vi "Create_empty_waveform_file.vi"(11 "File#":u8) -> (0 "error out":errorcluster)   [LabVIEW 2017]
uses:
  <vilib>/Waveform/WDTFileIO.llb/ Write Waveform to File.vi
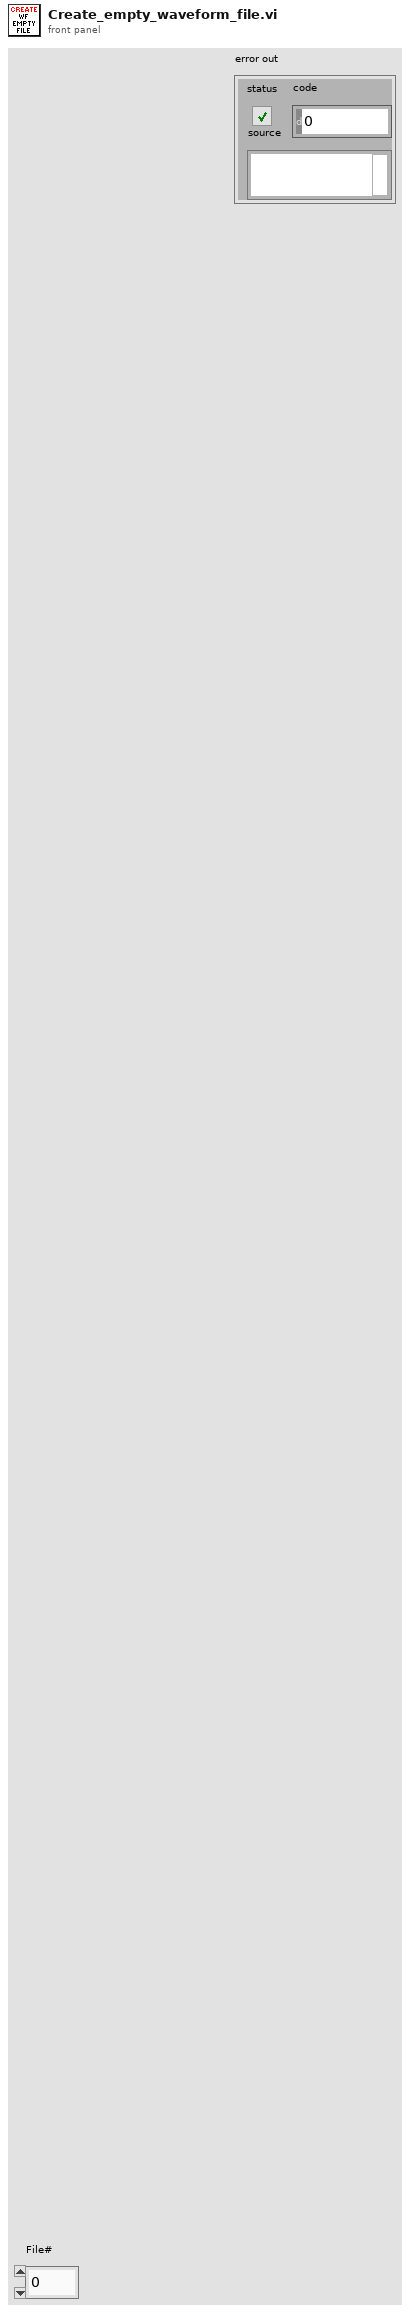
[diagram p1: front panel]
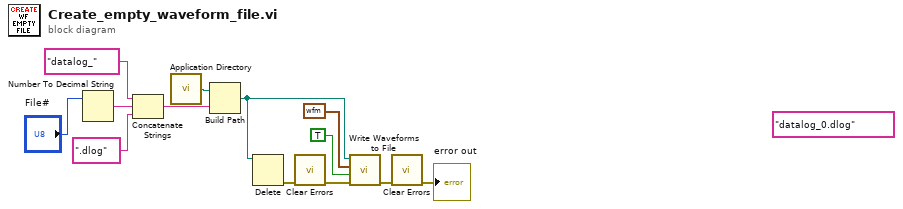
[diagram p0: block diagram]
diagram:
  (unwired) "datalog_0.dlog" ("pattern label")
  n1 = Number To Decimal String(number="File#") -> (decimal integer string=w4:string)  [unwired: 1 in]
  n2 = Concatenate Strings("datalog_" ("string"), w4, ".dlog" ("string")) -> (w3:string)
  n3 = call <vilib>:"Application Directory.vi"() -> ("Application Directory"=w6:path)
  n4 = Build Path(base path=w6, name or relative path=w3) -> (appended path=w11:path)
  n5 = Delete(path (use dialog)=w11) -> (error out=w9:errorcluster)  [unwired: 4 in, 2 out]
  n6 = call <vilib>:"Clear Errors.vi"("error in (no error)"=w9) -> ("error out"=w10:errorcluster)  [unwired: 5 in, 1 out]
  n7 = call-poly <vilib>:"Write Waveforms to File.vi"("error in (no error)"=w10, "append to file? (new file:F)"=TRUE, "waveform"=waveform(dbl) {"t0"=timestamp(0 s since 1904-01-01), "dt"=1.0, "Y"=[]}, "file path (dialog if empty)"=w11) -> ("error out"=w8:errorcluster)  [unwired: 6 in, 1 out]
  n8 = call <vilib>:"Clear Errors.vi"("error in (no error)"=w8) -> ("error out"=→"error out":errorcluster)  [unwired: 5 in, 1 out]
